vi "user.free.vi"(8 "error in":errorcluster, 11 "User in":refnum<class "User.lvclass">) -> (0 "error out":errorcluster)   [LabVIEW 2020, in "User.lvclass"]
doc: "Releases the handle and its associated resources."
uses:
  User.lvclass
  User.lvclass/User.ctl
  client.lvlib
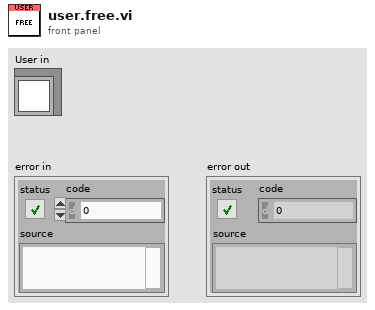
[diagram p1: front panel]
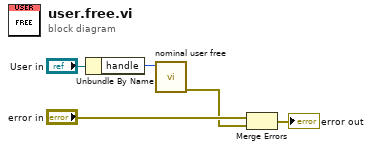
[diagram p0: block diagram]
diagram:
  n1 = Unbundle By Name("User in") -> ("handle"=w5:i32)
  n2 = call "nominal user free.vi"("user"=w5) -> ("error out"=w2:errorcluster)  [unwired: 9 in, 1 out]
  n3 = Merge Errors("error in", w2) -> (→"error out":errorcluster)
